vi "SR830-reserve.vi"(8 "error in (no error)":errorcluster, 10 "Dynamic Reserve (-1: Auto Reserve)":i16(ring)=-1 items=["Auto Reserve"=-1, "High Reserve"=0, "Normal"=1, "Low Noise"=2], 11 "VISA resource name":refnum<visa-resource-name>) -> (0 "error out":errorcluster, 3 "VISA resource name out":refnum<visa-resource-name>)   [LabVIEW 2019, in "User lib.lvlib"]
uses:
  User lib.lvlib
  lib/Stanford Research 830/Stanford Research 830.lvlib
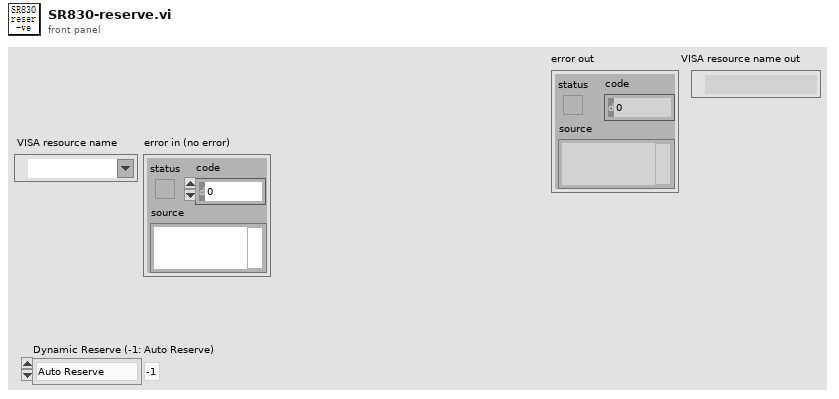
[diagram p1: front panel]
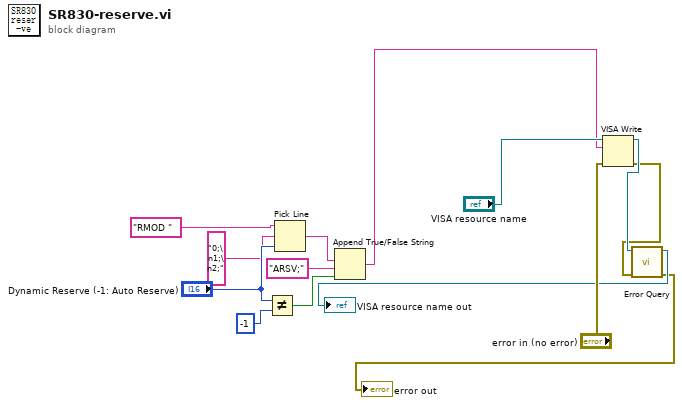
[diagram p0: block diagram]
diagram:
  n1 = Not Equal?(x="Dynamic Reserve (-1: Auto Reserve)", y=i16 -1) -> (x != y?=w8:bool)
  n2 = Pick Line(string ("")="RMOD ", multi-line string="0;\n1;\n2;", line index="Dynamic Reserve (-1: Auto Reserve)") -> (output string=w3:string)
  n3 = Append True/False String(1:w8, 2:"ARSV;" ("false string"), 3:w3) -> (0:w1:string)  [unwired: 1 in]
  n4 = VISA Write(VISA resource name="VISA resource name", write buffer=w1, error in (no error)="error in (no error)") -> (VISA resource name out=w14:refnum<visa-resource-name>, error out=w10:errorcluster)  [unwired: 1 out]
  n5 = call "Error Query.vi"("error in (no error)"=w10, "VISA resource name"=w14) -> ("error out"=→"error out":errorcluster, "VISA resource name out"=→"VISA resource name out":refnum<visa-resource-name>)  [unwired: 7 in, 1 out]
